vi "Create UI_main.vi"(7 "main_UI in":refnum<class "UI_main.lvclass">, 8 "error in (no error)":errorcluster, 10 "lockin":refnum<class "lockin.lvclass">) -> (0 "error out":errorcluster, 3 "main_UI out":refnum<class "UI_main.lvclass">)   [LabVIEW 2016, in "UI_main.lvclass"]
uses:
  UI_main.lvclass
  C:/Program Files (x86)/National Instruments/LabVIEW 2016/vi.lib/JKI/JKI SMO/SMO/SMO.lvclass
  lockin/lockin.lvclass
  UI_main.lvclass/UI_main.ctl
  <vilib>/JKI/JKI SMO/SMO/SMO.lvclass
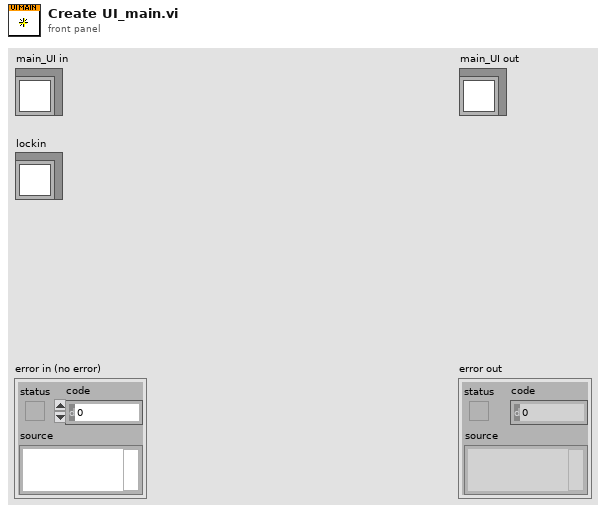
[diagram p1: front panel]
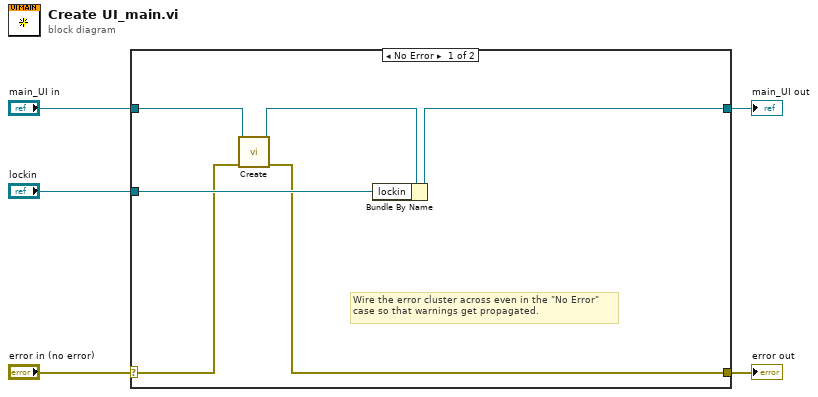
[diagram p0: block diagram]
diagram:
  n1 = case shown="No Error" "error in (no error)" {
    selector: "error in (no error)" -> [w7 w13]
    tunnel: [w6 w13] -> w4
    tunnel: [w10 w12] -> w2
    tunnel: "main_UI in" -> [w9 w12]
    tunnel: "lockin" -> [w11 _]
    frame No Error {
      # "Wire the error cluster across even in the \"No Error\"\ncase so that warnings get propagated."
      n2 = call <vilib>:"Create.vi"("error in (no error)"=w7, "SMO"=w9) -> ("error out"=w6:errorcluster, "SMO out"=w8:refnum<class "UI_main.lvclass">)  [unwired: 7 in, 1 out]
      n3 = Bundle By Name(cluster=w8, "lockin"=w11) -> (w10:refnum<class "UI_main.lvclass">)
    }
    frame Error {
    }
  }
  "error out" <- w4
  "main_UI out" <- w2
